vi "Move Impl.vi"(6 "Mode":enum16{"Relative", "Absolute"}(ring), 8 "error in (no error)":errorcluster, 9 "Value (mm)":dbl format="%#_13g", 10 "Axis":T1=enum."Y", 11 "Ludl Stage in":refnum<class "Ludl Stage.lvclass">) -> (0 "error out":errorcluster, 3 "Ludl Stage out":refnum<class "Ludl Stage.lvclass">)   [LabVIEW 2023, in "Ludl Stage.lvlib" / "Ludl Stage.lvclass"]
uses:
  Stage Controller/Stage Axis.ctl
  Ludl Stage.lvclass
  Ludl Stage.lvclass/Ludl Stage.ctl
  Stage Controller/Stage Controller.lvlib
  Resources/GLOBAL/GLOBAL Debug.vi
  Stage Controller/Stage Controller.lvclass
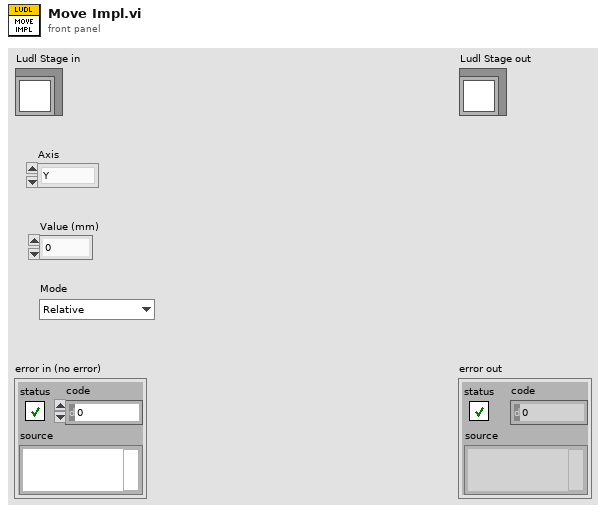
[diagram p1: front panel]
types:
  T1 = typedef "Stage Controller.lvlib/Stage Controller.lvclass/Stage Axis.ctl" = enum16{"unspecified", "X", "Y", "Z"}
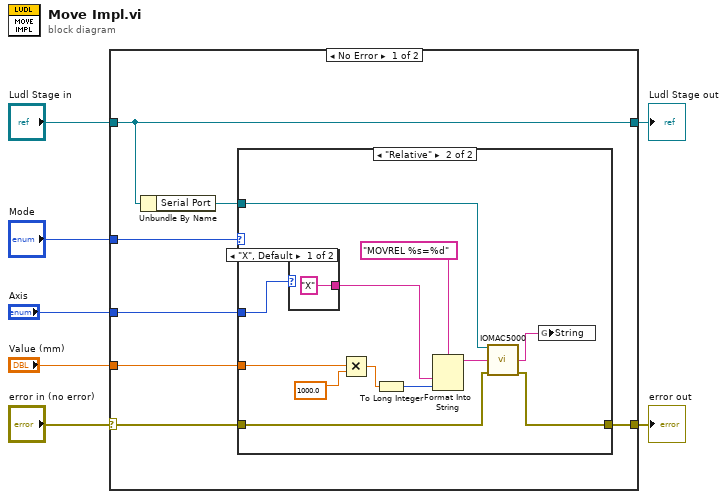
[diagram p0: block diagram]
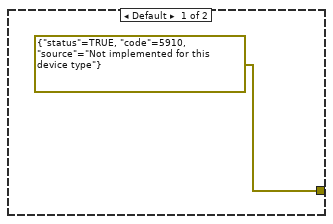
[diagram p2: hidden frame]
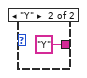
[diagram p3: hidden frame]
diagram:
  n1 = case shown="No Error" "error in (no error)" {
    selector: "error in (no error)" -> [w13 w31]
    tunnel: [w14 w31] -> w6
    tunnel: "Ludl Stage in" -> [w10 w30]
    tunnel: [w10 w30] -> w4
    tunnel: "Mode" -> [w8 _]
    tunnel: "Axis" -> [w12 _]
    tunnel: "Value (mm)" -> [w11 _]
    frame No Error {
      n2 = Unbundle By Name(w10) -> ("Serial Port"=w9:refnum<visa-resource-name>)
      n3 = case shown="\"Relative\"" w8 {
        tunnel: [errorcluster {"status"=TRUE, "code"=5910, "source"="Not implemented for this device type"} ("error IO") w21] -> w14
        tunnel: w13 -> [_ w20]
        tunnel: w12 -> [_ w19]
        tunnel: w11 -> [_ w17]
        tunnel: w9 -> [_ w16]
        frame Default {
        }
        frame "Relative" {
          n4 = case shown="\"X\", Default" w19 {
            tunnel: ["X" "Y"] -> w18
            frame "X", Default {
            }
            frame "Y" {
            }
          }
          n5 = Multiply(x=w17, y=1000.0) -> (x*y=w25:dbl)
          n6 = To Long Integer(number=w25) -> (32bit integer=w22:i32)
          n7 = Format Into String(format string="MOVREL %s=%d", w18, w22) -> (resulting string=w24:string)  [unwired: 2 in, 1 out]
          n8 = call "IOMAC5000.vi"("VISA  IN"=w16, "Command (to ctlr)"=w24, "error in"=w20) -> ("Raw Response"=w23:string, "error out"=w21:errorcluster)  [unwired: 9 in, 2 out]
          n9 = global write "GLOBAL Debug.vi" "String"(w23) -> ()
        }
      }
    }
    frame Error {
    }
  }
  "error out" <- w6
  "Ludl Stage out" <- w4
